vi "combo For-While Loop.vi"() -> ()   [LabVIEW 2018]
panel:
  in  "stop":bool
  out "Numeric 2":dbl
  in  "Numeric":dbl
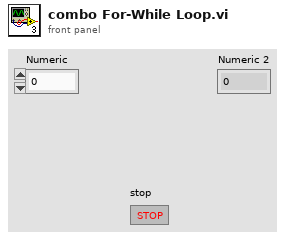
[diagram p1: front panel]
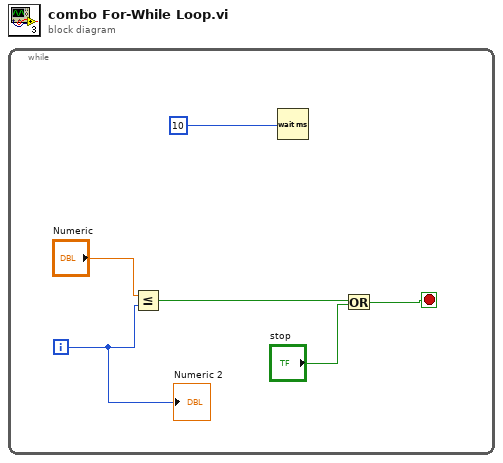
[diagram p0: block diagram]
diagram:
  n1 = while {
    i -> [w5]
    stop <- w3 stop-if-true
    n2 = Less Or Equal?(x="Numeric", y=w5) -> (x <= y?=w4:bool)
    n3 = Wait (ms)(milliseconds to wait=10) -> ()  [unwired: 1 out]
    n4 = Or(x=w4, y="stop") -> (x .or. y?=w3:bool)
    "Numeric 2" <- w5
  }
